vi "Terminal.vi"() -> ()   [LabVIEW 2014]
panel:
  out "数据采集":T1
  in  "P 2":u16
  in  "P":u16
  in  "T":u16
  in  "L":u16
  in  "陪试轴承润滑单元开关":bool
  in  "试验轴承润滑单元开关":bool
  in  "F2":u16
  in  "F1":u16
  in  "加载单元开关":bool
  out "齿轮子系统-PLC":u16[](graph)
  in  "齿轮子系统开关":bool
  out "动力子系统-PLC":u16[](graph)
  out "NI工控机":u16[](array[numeric])
  out "动力子系统-温度巡检仪":u16[](array[numeric])
  out "动力子系统-PLC":u16[](array[numeric])
  out "齿轮子系统-数显表":u16[](array[numeric])
  out "齿轮子系统-PLC":u16[](array[numeric])
  out "液压子系统":u16[](array[numeric])
  in  "电机转速":u16
  in  "动力子系统开关":bool
  out "error out":errorcluster caption="错误输出"
  in  "DAQ模块":bool
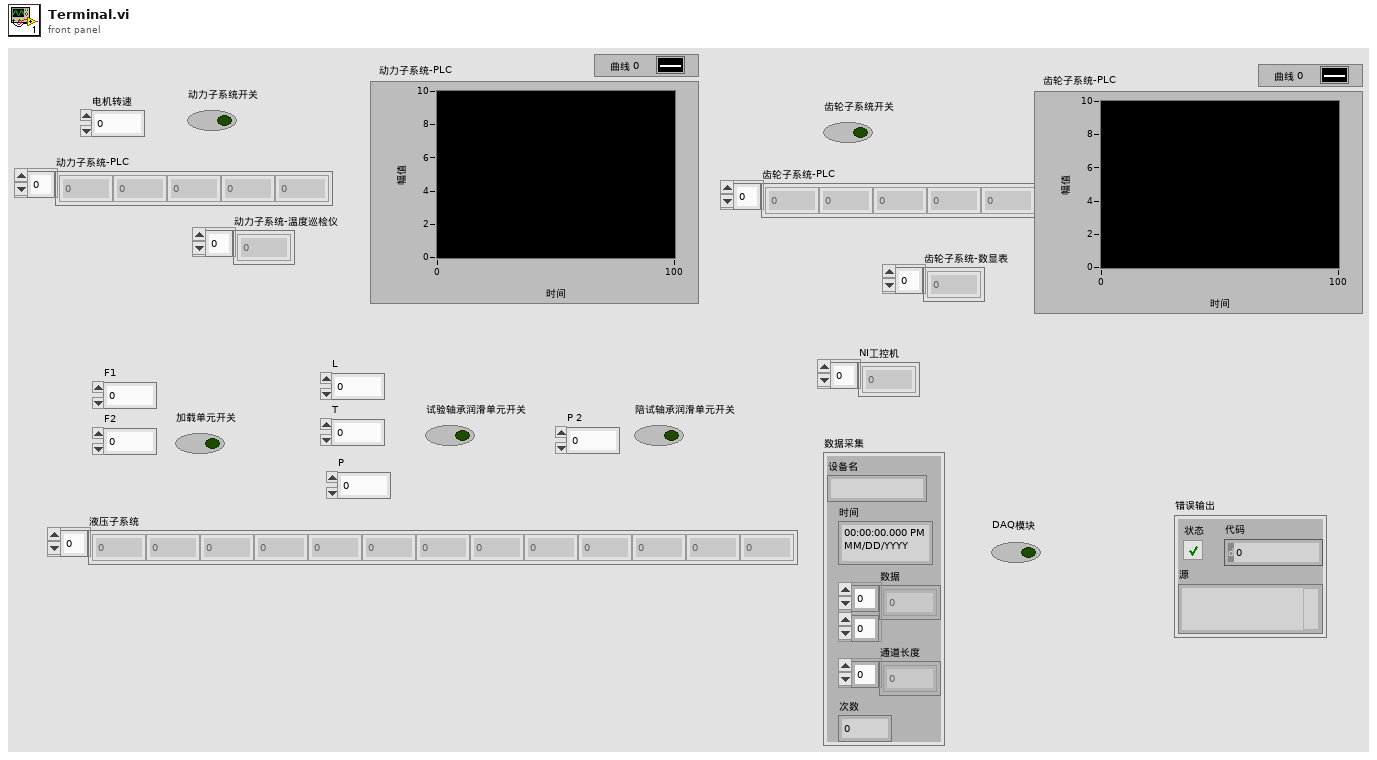
[diagram p1: front panel]
types:
  T1 = cluster{"设备名":string, "时间":timestamp, "数据":sgl[][], "通道长度":i32[], "次数":i32}
  T2 = cluster{"switch":bool, "L":u16, "T":u16, "P":u16}
  T3 = cluster{"Transaction ID":u16, "Unit ID":u8, "Starting Address":u16, "Quantity":u16, "Holding Registers":u16[], "Exception Code":u8}
  T4 = cluster{"Transaction ID":u16, "Unit ID":u8, "Address":u16, "Register":i32}
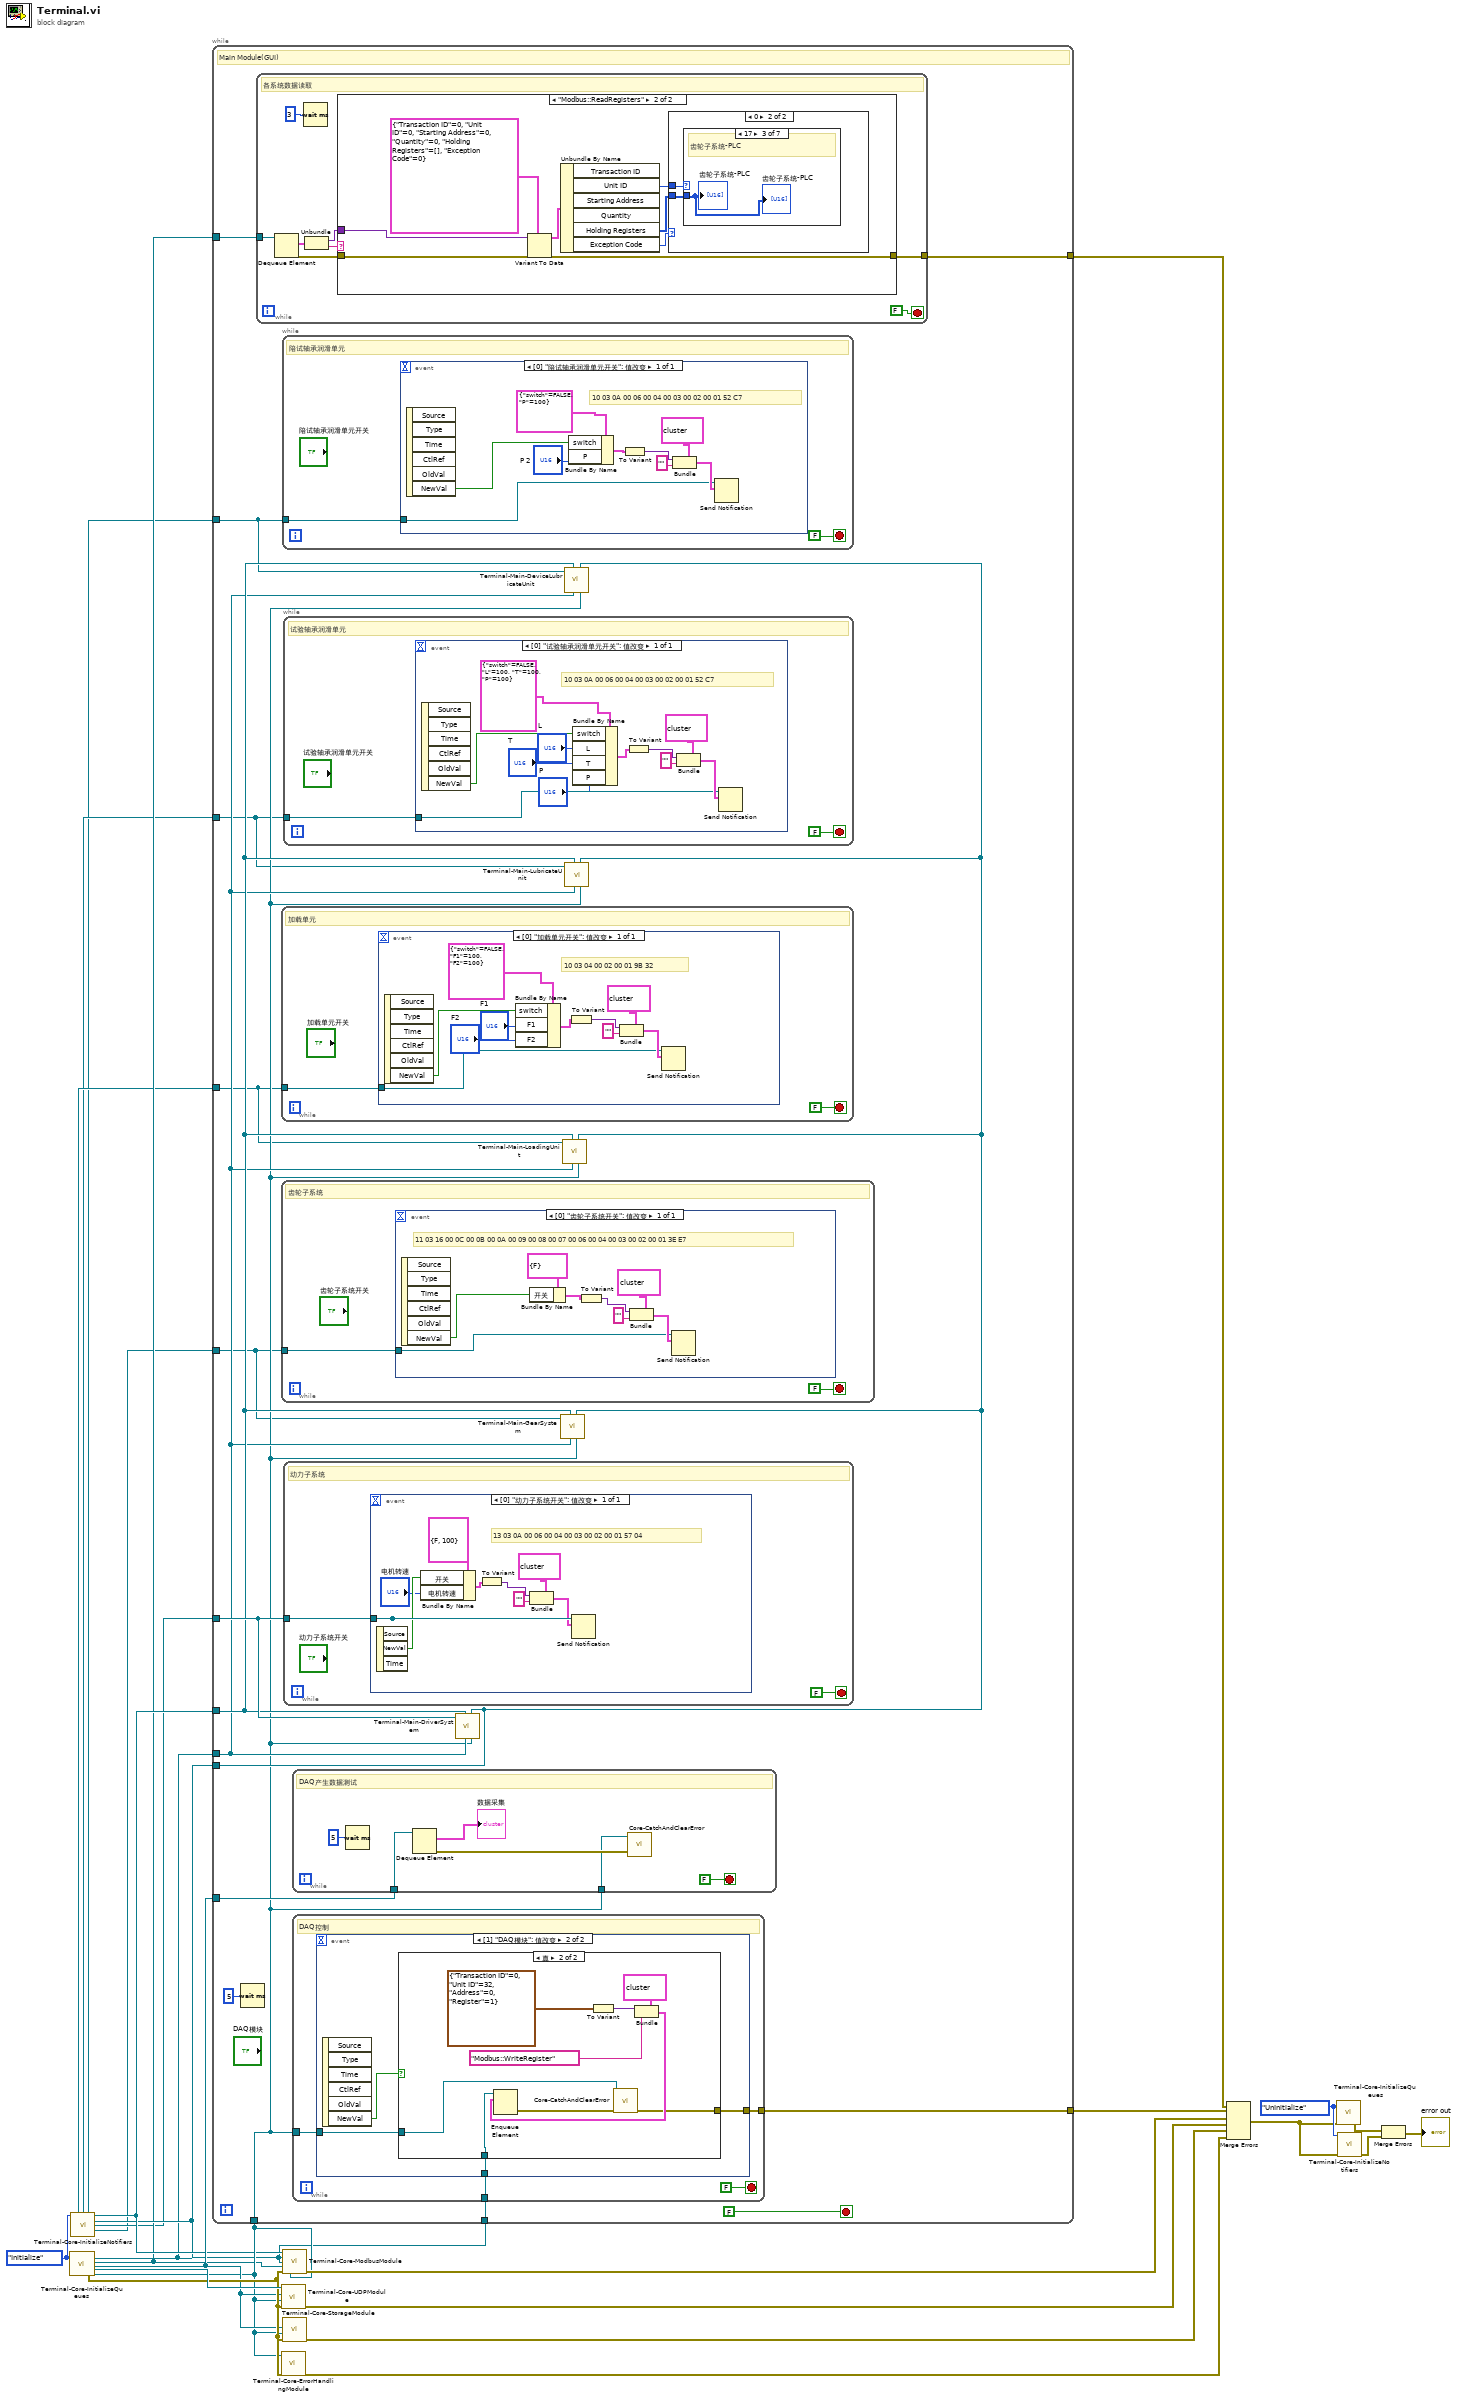
[diagram p0: block diagram]
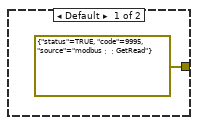
[diagram p2: hidden frame]
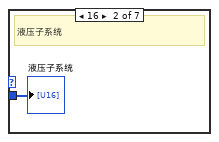
[diagram p5: hidden frame]
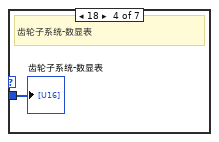
[diagram p6: hidden frame]
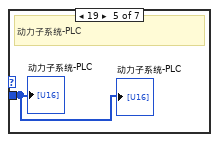
[diagram p7: hidden frame]
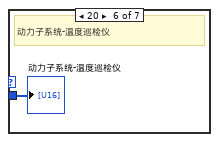
[diagram p8: hidden frame]
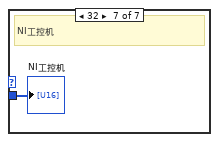
[diagram p9: hidden frame]
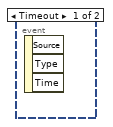
[diagram p10: hidden frame]
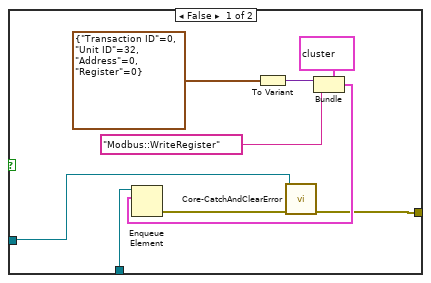
[diagram p11: hidden frame]
diagram:
  w17 = enum16{"UnInitialize", "Initialize"}."UnInitialize" ("comand (Initialize)")
  w18 = enum16{"UnInitialize", "Initialize"}."Initialize" ("comand (Initialize)")
  n1 = call "Terminal-Core-InitializeQueues.vi"("comand (Initialize)"=w18) -> ("error out"=w24:errorcluster, "ModbusMsgQRef"=w9:refnum<queue>, "GuiModbusQRef"=w8:refnum<queue>, "DataQRef"=w19:refnum<queue>, "UdpQRef"=w25:refnum<queue>, "ErrorQRef"=w12:refnum<queue>)  [unwired: 12 in, 1 out]
  n2 = call "Terminal-Core-InitializeNotifiers.vi"("comand (Initialize)"=w18) -> ("LoadingUnitNRef"=w3:refnum<notifier>, "LubricateUnitNRef"=w2:refnum<notifier>, "DeviceLubricateUnitNRef"=w1:refnum<notifier>, "ModbusNReqRef"=w11:refnum<notifier>, "ModbusNResRef"=w10:refnum<notifier>, "DriverSystemNRef"=w5:refnum<notifier>, "GearSystemNRef"=w4:refnum<notifier>)  [unwired: 7 in, 1 out]
  n3 = while {
    tunnel: w9 -> [w39]
    tunnel: w12 -> [w30]
    tunnel: [w38] -> w7
    tunnel: w19 -> [w37]
    tunnel: w11 -> [w32]
    tunnel: w10 -> [w33]
    tunnel: w9 -> [w31]
    tunnel: w5 -> [w36]
    tunnel: w8 -> [w35]
    tunnel: [w34] -> w6
    tunnel: w4 -> [w29]
    tunnel: w3 -> [w28]
    tunnel: w2 -> [w27]
    tunnel: w1 -> [w26]
    stop <- FALSE stop-if-true
    # "Main Module(GUI)"
    n4 = Wait (ms)(milliseconds to wait=u32 5 ("等待时间（毫秒）")) -> ()  [unwired: 1 out]
    n5 = while {
      tunnel: w35 -> [w95]
      tunnel: [w90] -> w34
      stop <- FALSE stop-if-true
      # "各系统数据读取"
      n6 = Dequeue Element(queue=w95) -> (element=w94:cluster{variant, string}, error out=w91:errorcluster)  [unwired: 2 in, 2 out]
      n7 = Wait (ms)(milliseconds to wait=u32 3 ("等待时间（毫秒）")) -> ()  [unwired: 1 out]
      n8 = Unbundle(w94) -> (w92:variant, w93:string)
      n9 = case shown="\"Modbus::ReadRegisters\"" w93 {
        tunnel: w92 -> [_ w104]
        tunnel: w91 -> [_ w103]
        tunnel: [errorcluster {"status"=TRUE, "code"=9995, "source"="modbus：：GetRead"} ("错误常量") w98] -> w90
        frame Default {
        }
        frame "Modbus::ReadRegisters" {
          n10 = Variant To Data(error in=w103, type=T3 {"Transaction ID"=0, "Unit ID"=0, "Starting Address"=0, "Quantity"=0, "Holding Registers"=[], "Exception Code"=0} ("元素"), Variant=w104) -> (data=w102:T3, error out=w98:errorcluster)
          n11 = Unbundle By Name(w102) -> ("Unit ID"=w99:u8, "Holding Registers"=w97:u16[], "Exception Code"=w100:u8)  [unwired: 3 out]
          n12 = case shown="0" w100 {
            tunnel: w99 -> [_ w106]
            tunnel: w97 -> [_ w105]
            frame Default {
            }
            frame 0 {
              n13 = case shown="17" w106 {
                tunnel: w105 -> [_ w107 w108 w109 w110 w111 w112]
                frame Default {
                }
                frame 16 {
                  # "液压子系统"
                  "液压子系统" <- w107
                }
                frame 17 {
                  # "齿轮子系统-PLC"
                  "齿轮子系统-PLC" <- w108
                  "齿轮子系统-PLC" <- w108
                }
                frame 18 {
                  # "齿轮子系统-数显表"
                  "齿轮子系统-数显表" <- w109
                }
                frame 19 {
                  # "动力子系统-PLC"
                  "动力子系统-PLC" <- w110
                  "动力子系统-PLC" <- w110
                }
                frame 20 {
                  # "动力子系统-温度巡检仪"
                  "动力子系统-温度巡检仪" <- w111
                }
                frame 32 {
                  # "NI工控机"
                  "NI工控机" <- w112
                }
              }
            }
          }
        }
      }
    }
    n14 = while {
      tunnel: w28 -> [w66]
      stop <- FALSE stop-if-true
      # "加载单元"
      n15 = event shown="[0] \"加载单元开关\": 值改变" {
        selector: _ -> [_]
        dyn-events: _ -> [_]
        timeout: _ -> [_]
        tunnel: w66 -> [w72]
        event "加载单元开关": Value Change {
          # "10 03 04 00 02 00 01 9B 32"
          n16 = event-data() -> ("NewVal"=w71:bool)  [unwired: 1 in, 5 out]
          n17 = Bundle By Name(cluster=cluster{"switch":bool, "F1":u16, "F2":u16} {"switch"=FALSE, "F1"=100, "F2"=100}, "switch"=w71, "F1"="F1", "F2"="F2") -> (w75:cluster{"switch":bool, "F1":u16, "F2":u16})
          n18 = To Variant(anything=w75) -> (Variant=w74:variant)
          n19 = Bundle(cluster=cluster{variant, string} {variant, ""}, w74, "") -> (w73:cluster{variant, string})
          n20 = Send Notification(notification=w73, notifier=w72) -> ()  [unwired: 1 in, 2 out]
        }
      }
    }
    n21 = while {
      tunnel: w29 -> [w79]
      stop <- FALSE stop-if-true
      # "齿轮子系统"
      n22 = event shown="[0] \"齿轮子系统开关\": 值改变" {
        selector: _ -> [_]
        dyn-events: _ -> [_]
        timeout: _ -> [_]
        tunnel: w79 -> [w80]
        event "齿轮子系统开关": Value Change {
          # "11 03 16 00 0C 00 0B 00 0A 00 09 00 08 00 07 00 06 00 04 00 03 00 02 00 01 3E E7"
          n23 = event-data() -> ("NewVal"=w81:bool)  [unwired: 1 in, 5 out]
          n24 = Bundle By Name(cluster=cluster{"开关":bool} {"开关"=FALSE}, "开关"=w81) -> (w84:cluster{"开关":bool})
          n25 = To Variant(anything=w84) -> (Variant=w83:variant)
          n26 = Bundle(cluster=cluster{variant, string} {variant, ""}, w83, "") -> (w82:cluster{variant, string})
          n27 = Send Notification(notification=w82, notifier=w80) -> ()  [unwired: 1 in, 2 out]
        }
      }
    }
    n28 = while {
      tunnel: w26 -> [w42]
      stop <- FALSE stop-if-true
      # "陪试轴承润滑单元"
      n29 = event shown="[0] \"陪试轴承润滑单元开关\": 值改变" {
        selector: _ -> [_]
        dyn-events: _ -> [_]
        timeout: _ -> [_]
        tunnel: w42 -> [w47]
        event "陪试轴承润滑单元开关": Value Change {
          # "10 03 0A 00 06 00 04 00 03 00 02 00 01 52 C7"
          n30 = event-data() -> ("NewVal"=w46:bool)  [unwired: 1 in, 5 out]
          n31 = Bundle By Name(cluster=cluster{"switch":bool, "P":u16} {"switch"=FALSE, "P"=100}, "switch"=w46, "P"="P 2") -> (w50:cluster{"switch":bool, "P":u16})
          n32 = To Variant(anything=w50) -> (Variant=w49:variant)
          n33 = Bundle(cluster=cluster{variant, string} {variant, ""}, w49, "") -> (w48:cluster{variant, string})
          n34 = Send Notification(notification=w48, notifier=w47) -> ()  [unwired: 1 in, 2 out]
        }
      }
    }
    n35 = while {
      tunnel: w27 -> [w53]
      stop <- FALSE stop-if-true
      # "试验轴承润滑单元"
      n36 = event shown="[0] \"试验轴承润滑单元开关\": 值改变" {
        selector: _ -> [_]
        dyn-events: _ -> [_]
        timeout: _ -> [_]
        tunnel: w53 -> [w59]
        event "试验轴承润滑单元开关": Value Change {
          # "10 03 0A 00 06 00 04 00 03 00 02 00 01 52 C7"
          n37 = event-data() -> ("NewVal"=w60:bool)  [unwired: 1 in, 5 out]
          n38 = Bundle By Name(cluster=T2 {"switch"=FALSE, "L"=100, "T"=100, "P"=100}, "switch"=w60, "L"="L", "T"="T", "P"="P") -> (w63:T2)
          n39 = To Variant(anything=w63) -> (Variant=w62:variant)
          n40 = Bundle(cluster=cluster{variant, string} {variant, ""}, w62, "") -> (w61:cluster{variant, string})
          n41 = Send Notification(notification=w61, notifier=w59) -> ()  [unwired: 1 in, 2 out]
        }
      }
    }
    n42 = while {
      tunnel: w36 -> [w113]
      stop <- FALSE stop-if-true
      # "动力子系统"
      n43 = event shown="[0] \"动力子系统开关\": 值改变" {
        selector: _ -> [_]
        dyn-events: _ -> [_]
        timeout: _ -> [_]
        tunnel: [w123] -> _
        tunnel: w113 -> [w123]
        event "动力子系统开关": Value Change {
          # "13 03 0A 00 06 00 04 00 03 00 02 00 01 57 04"
          n44 = event-data() -> ("NewVal"=w119:bool)  [unwired: 1 in, 2 out]
          n45 = Bundle By Name(cluster=cluster{"开关":bool, "电机转速":u16} {"开关"=FALSE, "电机转速"=100}, "开关"=w119, "电机转速"="电机转速") -> (w117:cluster{"开关":bool, "电机转速":u16})
          n46 = To Variant(anything=w117) -> (Variant=w116:variant)
          n47 = Bundle(cluster=cluster{variant, string} {variant, ""}, w116, "") -> (w115:cluster{variant, string})
          n48 = Send Notification(notification=w115, notifier=w123) -> ()  [unwired: 1 in, 2 out]
        }
      }
    }
    n49 = while {
      tunnel: w37 -> [w153]
      tunnel: w30 -> [w151]
      stop <- FALSE stop-if-true
      # "DAQ产生数据测试"
      n50 = Wait (ms)(milliseconds to wait=u32 5 ("等待时间（毫秒）")) -> ()  [unwired: 1 out]
      n51 = Dequeue Element(queue=w153) -> (element=→"数据采集":T1, error out=w152:errorcluster)  [unwired: 2 in, 2 out]
      n52 = call "Core-CatchAndClearError.vi"("error in (no error)"=w152, "ErrorQ"=w151) -> ()  [unwired: 7 in, 1 out]
    }
    n53 = while {
      tunnel: w39 -> [w127]
      tunnel: [w126] -> w38
      tunnel: w30 -> [w125]
      stop <- FALSE stop-if-true
      # "DAQ控制"
      n54 = event shown="[1] \"DAQ模块\": 值改变" {
        selector: _ -> [_ _]
        dyn-events: _ -> [_ _]
        timeout: _ -> [_ _]
        tunnel: w127 -> [_ w130]
        tunnel: w125 -> [_ w129]
        tunnel: [_ w128] -> w126
        event Timeout {
          n55 = event-data() -> ()  [unwired: 1 in, 3 out]
        }
        event "DAQ模块": Value Change {
          n56 = event-data() -> ("NewVal"=w131:bool)  [unwired: 1 in, 5 out]
          n57 = case shown="真" w131 {
            tunnel: w130 -> [w134 w142]
            tunnel: w129 -> [w133 w141]
            tunnel: [w135 w143] -> w128
            frame False {
              n58 = To Variant(anything=T4 {"Transaction ID"=0, "Unit ID"=32, "Address"=0, "Register"=0}) -> (Variant=w138:variant)
              n59 = Bundle(cluster=cluster{variant, string} {variant, ""}, w138, "Modbus::WriteRegister") -> (w137:cluster{variant, string})
              n60 = Enqueue Element(queue=w134, element=w137) -> (error out=w140:errorcluster)  [unwired: 2 in, 2 out]
              n61 = call "Core-CatchAndClearError.vi"("error in (no error)"=w140, "ErrorQ"=w133) -> ("error out"=w135:errorcluster)  [unwired: 7 in]
            }
            frame True {
              n62 = To Variant(anything=T4 {"Transaction ID"=0, "Unit ID"=32, "Address"=0, "Register"=1}) -> (Variant=w147:variant)
              n63 = Bundle(cluster=cluster{variant, string} {variant, ""}, w147, "Modbus::WriteRegister") -> (w146:cluster{variant, string})
              n64 = Enqueue Element(queue=w142, element=w146) -> (error out=w149:errorcluster)  [unwired: 2 in, 2 out]
              n65 = call "Core-CatchAndClearError.vi"("error in (no error)"=w149, "ErrorQ"=w141) -> ("error out"=w143:errorcluster)  [unwired: 7 in]
            }
          }
        }
      }
    }
    n66 = call "Terminal-Main-DriverSystem.vi"("ErrorQRef"=w30, "ModbusNResRef"=w33, "ModbusMsgQRef"=w31, "ModbusNReqRef"=w32, "DriverSystemNRef"=w36) -> ()  [unwired: 6 in, 1 out]
    n67 = call "Terminal-Main-GearSystem.vi"("ErrorQRef"=w30, "ModbusNResRef"=w33, "ModbusMsgQRef"=w31, "ModbusNReqRef"=w32, "GearSystemNRef"=w29) -> ()  [unwired: 6 in, 1 out]
    n68 = call "Terminal-Main-LoadingUnit.vi"("ErrorQRef"=w30, "ModbusNResRef"=w33, "ModbusMsgQRef"=w31, "ModbusNReqRef"=w32, "LoadingUnitNRef"=w28) -> ()  [unwired: 6 in, 1 out]
    n69 = call "Terminal-Main-DeviceLubricateUnit.vi"("ErrorQRef"=w30, "ModbusNResRef"=w33, "ModbusMsgQRef"=w31, "ModbusNReqRef"=w32, "DeviceLubricateUnitNRef"=w26) -> ()  [unwired: 6 in, 1 out]
    n70 = call "Terminal-Main-LubricateUnit.vi"("ErrorQRef"=w30, "ModbusNResRef"=w33, "ModbusMsgQRef"=w31, "ModbusNReqRef"=w32, "LubricateUnitNRef"=w27) -> ()  [unwired: 6 in, 1 out]
  }
  n71 = call "Terminal-Core-UDPModule.vi"("error in"=w24, "ErrorQRef"=w12, "DataQRef"=w19, "UdpQRef"=w25) -> ("错误输出"=w21:errorcluster)  [unwired: 7 in]
  n72 = call "Terminal-Core-ErrorHandlingModule.vi"("error in"=w24, "ErrorQRef"=w12) -> ("error out"=w23:errorcluster)  [unwired: 9 in]
  n73 = call "Terminal-Core-ModbusModule.vi"("ModbusNReqRef"=w11, "ModbusNResRef"=w10, "ModbusMsgQRef"=w9, "GuiModbusQRef"=w8, "error in"=w24, "ErrorQRef"=w12) -> ("error out"=w20:errorcluster)  [unwired: 9 in]
  n74 = call "Terminal-Core-StorageModule.vi"("error in"=w24, "ErrorQRef"=w12, "DataQRef"=w19) -> ("错误输出"=w22:errorcluster)  [unwired: 8 in]
  n75 = Merge Errors(w6, w7, w20, w21, w22, w23) -> (w16:errorcluster)
  n76 = call "Terminal-Core-InitializeQueues.vi"("comand (Initialize)"=w17, "error in (no error)"=w16) -> ("error out"=w14:errorcluster)  [unwired: 11 in, 6 out]
  n77 = call "Terminal-Core-InitializeNotifiers.vi"("comand (Initialize)"=w17, "error in (no error)"=w16) -> ("error out"=w15:errorcluster)  [unwired: 6 in, 7 out]
  n78 = Merge Errors(w14, w15) -> (→"error out":errorcluster)
